vi "ManipActuateHopper.vi"(2 "Reinit":bool, 3 "Parameter String":string) -> (0 "error out":errorcluster, 1 "Advance Trigger":bool)   [LabVIEW 2020]
doc: "This VI commands the hopper to open or close during a systems check\n\nParameters:\nDecides open or closed state of the hopper (\"open\" or \"close\")"
uses:
  SafeParser_String.vi
  GlobalDriverStationCommands.vi
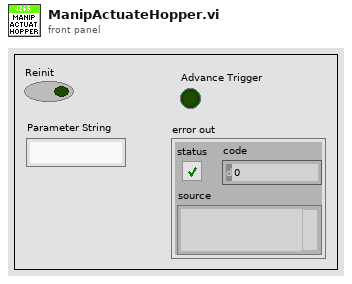
[diagram p1: front panel]
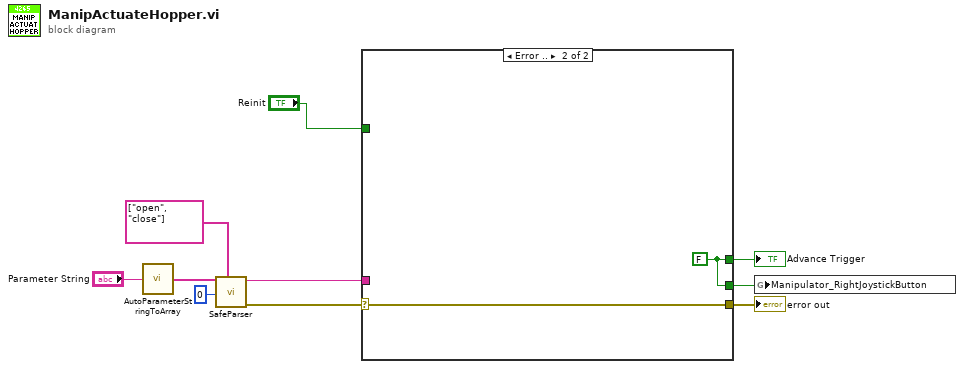
[diagram p0: block diagram]
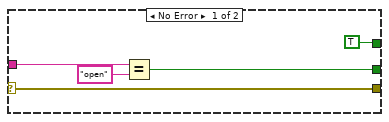
[diagram p2: hidden frame]
diagram:
  n1 = call "AutoParameterStringToArray.vi"("Parameter String"="Parameter String") -> ("Parsed Parameters"=w8:string[])
  n2 = call-poly "SafeParser.vi"("Allowed Values"=string[] ["open", "close"], "Array Index"=0 ("Parameter Index"), "String Array"=w8) -> ("Error Out"=w6:errorcluster, "Typecast Value"=w3:string)  [unwired: 7 in]
  n3 = case shown="Error .." w6 {
    selector: w6 -> [w15 w17]
    tunnel: [w13 w16] -> w1
    tunnel: [w15 w17] -> w5
    tunnel: "Reinit" -> [_ _]
    tunnel: w3 -> [w14 _]
    tunnel: [TRUE w16] -> w2
    frame No Error {
      n4 = Equal?(x=w14, y="open") -> (x = y?=w13:bool)
    }
    frame Error {
      w16 = FALSE
    }
  }
  "Advance Trigger" <- w2
  "error out" <- w5
  n5 = global write "GlobalDriverStationCommands.vi" "Manipulator_RightJoystickButton"(w1) -> ()
